vi "Stack2Montage.vi"(10 "Columns":i32=15, 11 "StackedAvg":u16[][][](array[numeric])=array210x120x120[3024000 elements]) -> (2 "ColorScale":picture, 3 "Montage":picture)   [LabVIEW 2014]
uses:
  <vilib>/picture/picture.llb/Draw True-Color Pixmap.vi
  ColorMaps.ctl
panel:
  in  "ColorMap":T1=59 items=["Bathymetry9", "BlackBody", "Blue", "BlueBlackRed", "BlueGreenOrange", "BlueHot", "BlueHot256", "BlueRedGreen", "BlueRedGreen256", "BrownViolet", "Classification", "ColdWarm", "Copper", "Cyan", "CyanMagenta", "Cycles", "dBZ14", "dBZ21", "EOSOrangeBlue11", "EOSSpectral11", "Fiddle", "Geo", "Geo32", "Gold", "Grays", "Grays16", "Grays256", "Green", "GreenMagenta16", "LandAndSea", "LandAndSea8", "Magenta", "Mocha", "Mud", "Pastels", "PastelsMap", "PastelsMap20", "PlanetEarth", "PlanetEarth256", "Rainbow", "Rainbow4Cycles", "Rainbow16", "Rainbow256", "RainbowCycle", "Red", "RedWhiteBlue", "RedWhiteBlue256", "RedWhiteGreen", "Relief", "Relief19", "SeaLandAndFire", "Spectrum", "SpectrumBlack", "Terrain", "Terrain256", "VioletOrangeYellow", "Web216", "Yellow", "YellowHot", "YellowHot256"]
  in  "Low":dbl
  in  "High":dbl=255.0
  in  "SpacePix":i32=2
  out "Sizes":i32[](array[numeric])=[210, 120, 120]
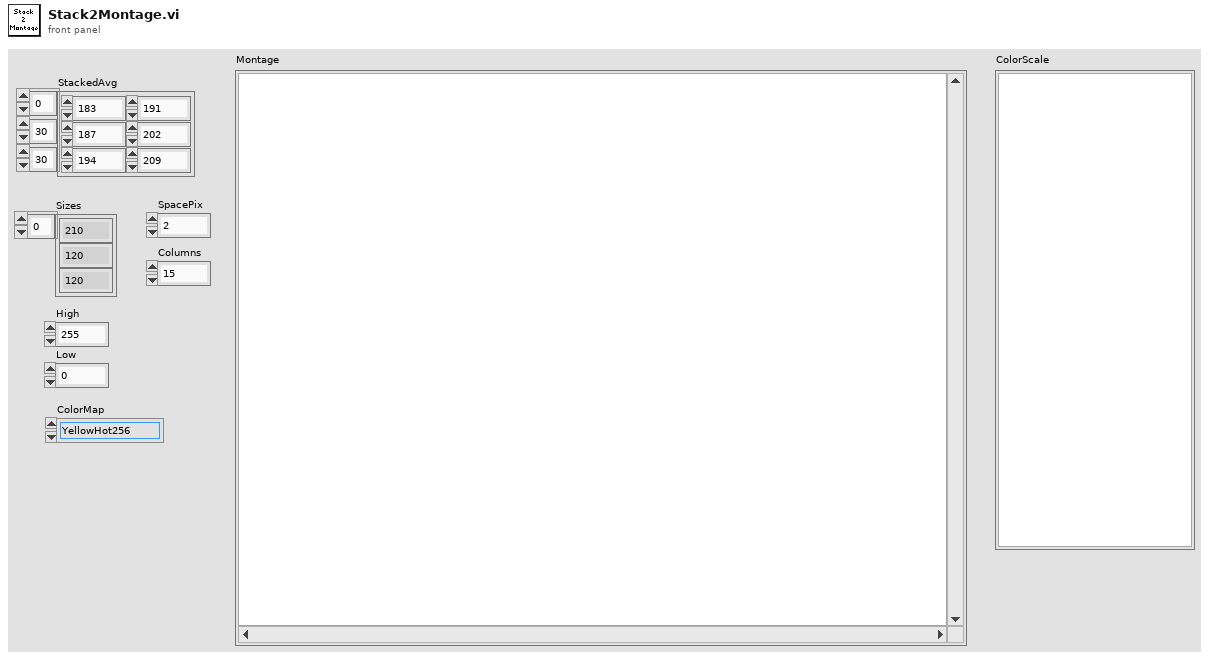
[diagram p1: front panel]
types:
  T1 = typedef "ColorMaps.ctl" = u16
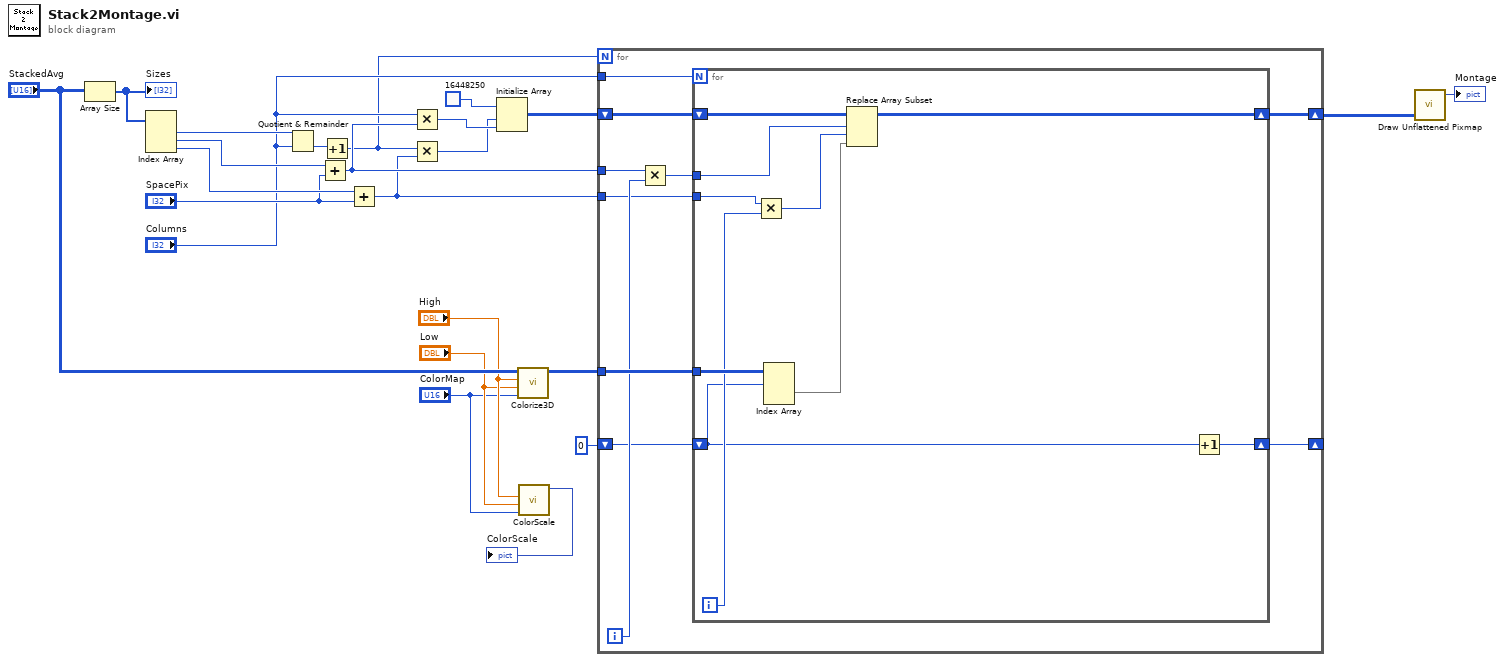
[diagram p0: block diagram]
diagram:
  n1 = Array Size(array="StackedAvg") -> (size(s)=w23:i32[])
  "Sizes" <- w23
  n2 = Index Array(array=w23) -> (element #1=w22:i32, element #2=w21:i32, element #3=w20:i32)  [unwired: 3 in]
  n3 = Quotient & Remainder(x=w22, y="Columns") -> (floor(x/y)=w11:i32)  [unwired: 1 out]
  n4 = Add(x=w21, y="SpacePix") -> (x+y=w16:i32)
  n5 = Increment(x=w11) -> (x+1=w7:i32)
  n6 = Add(x=w20, y="SpacePix") -> (x+y=w10:i32)
  n7 = Multiply(x="Columns", y=w16) -> (x*y=w6:i32)
  n8 = Multiply(x=w7, y=w10) -> (x*y=w5:i32)
  n9 = Initialize Array(u32 16448250, w5, w6) -> (w17:u32[][])
  n10 = call "Colorize3D.vi"("ColorMap"="ColorMap", "Low"="Low", "High"="High", "StackIn"="StackedAvg") -> ("Colorized"=w15:u32[][][])  [unwired: 7 in]
  n11 = call "ColorScale.vi"("ColorMap"="ColorMap", "Low"="Low", "High"="High") -> ("ColorScale"=→"ColorScale":picture)  [unwired: 8 in]
  n12 = for {
    N: w7 -> [_]
    shift-right: [w29] -> w13
    shift-left: w17 -> [w33]
    tunnel: w16 -> [w32]
    tunnel: w15 -> [w31]
    tunnel: w10 -> [w27]
    shift-right: [w25] -> _
    shift-left: 0 -> [w26]
    tunnel: "Columns" -> [w24]
    i -> [w30]
    n13 = Multiply(x=w32, y=w30) -> (x*y=w28:i32)
    n14 = for {
      N: w24 -> [_]
      tunnel: w31 -> [w42]
      tunnel: w28 -> [w34]
      tunnel: w27 -> [w40]
      shift-right: [w41] -> w29
      shift-left: w33 -> [w43]
      shift-right: [w36] -> w25
      shift-left: w26 -> [w37]
      i -> [w39]
      n15 = Multiply(x=w40, y=w39) -> (x*y=w35:i32)
      n16 = Index Array(array=w42, index (dim 0)=w37) -> (element=w38:u32[][])  [unwired: 2 in]
      n17 = Replace Array Subset(array=w43, new element=w38, index (row)=w34, index (col)=w35) -> (w41:u32[][])
      n18 = Increment(x=w37) -> (x+1=w36:i32)
    }
  }
  n19 = call-poly <vilib>:"Draw Unflattened Pixmap.vi"("data (RGB format)"=w13) -> ("new picture"=→"Montage":picture)  [unwired: 8 in]
